vi "lqSetManifestation.vi"(8 "error in (no error)":errorcluster, 10 "Manifestation":u32, 11 "QObject in":refnum<class "QObject.lvclass">) -> (0 "error out":errorcluster, 3 "QObject out":refnum<class "QObject.lvclass">)   [LabVIEW 2013, in "Template.lvlib" / "QObject.lvclass"]
uses:
  QObject.lvclass
  QObject.lvclass/QObject.ctl
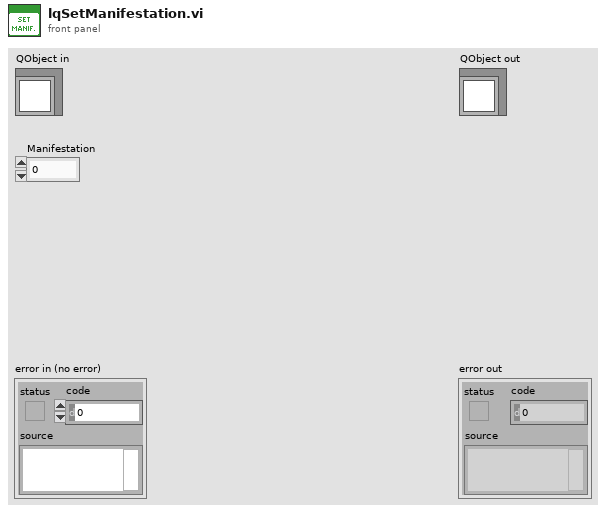
[diagram p1: front panel]
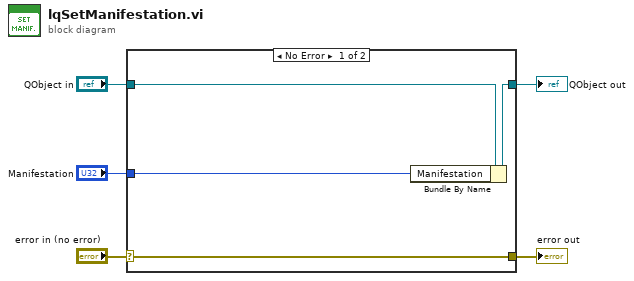
[diagram p0: block diagram]
diagram:
  n1 = case shown="No Error" "error in (no error)" {
    selector: "error in (no error)" -> [w9 w10]
    tunnel: [w9 w10] -> w4
    tunnel: [w7 w11] -> w2
    tunnel: "QObject in" -> [w8 w11]
    tunnel: "Manifestation" -> [w6 _]
    frame No Error {
      n2 = Bundle By Name(cluster=w8, "Manifestation"=w6) -> (w7:refnum<class "QObject.lvclass">)
    }
    frame Error {
    }
  }
  "error out" <- w4
  "QObject out" <- w2
